vi "Actor Core.vi"(8 "error in":errorcluster caption="错误输入", 11 "Input Operator in":refnum<class "ControlPanel.lvclass"> caption="操作者输入") -> (0 "error out":errorcluster caption="错误输出", 3 "操作者输出":refnum<class "Actor.lvclass">)   [LabVIEW 2014, in "ControlPanel.lvlib" / "ControlPanel.lvclass"]
doc: "(<B>文件名</B>：Actor Framework.lvlib:Actor.lvclass:Actor Core.vi)\n\n接收发送至操作者的消息，响应消息并处理可能导致操作者关闭的错误。\n\n子孙类重写该VI，使操作者完成特定的任务。使用调用父方法节点实现重写。"
uses:
  ControlPanel.lvclass
  <vilib>/ActorFramework/Actor/Actor.lvclass
  ctl/XBOX_Control.ctl
  <vilib>/MakerHub/Xbox-One-Controller/Private/Type Defs/Indicators/All Buttons Visual.ctl
  <vilib>/MakerHub/Xbox-One-Controller/Private/Type Defs/Indicators/A.ctl
  <vilib>/MakerHub/Xbox-One-Controller/Private/Type Defs/Indicators/B.ctl
  <vilib>/MakerHub/Xbox-One-Controller/Private/Type Defs/Indicators/X.ctl
  <vilib>/MakerHub/Xbox-One-Controller/Private/Type Defs/Indicators/Y.ctl
  <vilib>/MakerHub/Xbox-One-Controller/Private/Type Defs/Indicators/Left Bumper.ctl
  <vilib>/MakerHub/Xbox-One-Controller/Private/Type Defs/Indicators/Right Bumper.ctl
  <vilib>/MakerHub/Xbox-One-Controller/Private/Type Defs/Indicators/View.ctl
  <vilib>/MakerHub/Xbox-One-Controller/Private/Type Defs/Indicators/Menu.ctl
  <vilib>/MakerHub/Xbox-One-Controller/Private/Type Defs/Indicators/Thumbstick.ctl
  <vilib>/MakerHub/Xbox-One-Controller/Private/Type Defs/Indicators/All Axis Data.ctl
  <vilib>/MakerHub/Xbox-One-Controller/Private/Type Defs/Indicators/DPad Enum.ctl
  ctl/P3AT_InputCMD.ctl
  ctl/P3AT_Panel.ctl
  ctl/Actor_Control.ctl
  ctl/Semantic_Voice_Array.ctl
  ctl/P3AT_Ini_Pose_send_return.ctl
  JoyStick_lib/JoyStick/JoyStick.lvclass
  Dialogue_lib/DialogueActor/Dialogue.lvclass
  <vilib>/ActorFramework/Actor/Actor.lvclass/Actor.ctl
  <vilib>/ActorFramework/Message Enqueuer/Message Enqueuer.lvclass/Message Enqueuer.ctl
  ControlPanel.lvclass/ControlPanel.ctl
  <vilib>/ActorFramework/Message Enqueuer/Init from Existing Queue.vi
  <vilib>/ActorFramework/Message Enqueuer/Enqueue.vi
  Global_var/Global_var.vi
  <vilib>/ActorFramework/Message Priority Queue/Priority Enqueue.vi
  <vilib>/ActorFramework/Message Enqueuer/Message Enqueuer.lvclass
  Voice_lib/VoiceControl/Voice.lvclass
  <vilib>/ActorFramework/Stop Msg/Stop Msg.lvclass
  Wrapper_lib/zsActor/ActorWrapper.lvclass
  <vilib>/MakerHub/Xbox-One-Controller/LMH-Xbox-One-Controller.lvlib
panel:
  out "Semantic_DialoguePYPL_Array":T1
  out "Semantic_Dialogue_Array":T1
  out "Global_Planner_Recyle":bool
  in  "手动定位":T2
  out "Semantic_Voice_Array":T1
  out "P3AT_InputCMD":T3
  out "XBOX_Control":T4
  out "事件记录":string
  out "sensor":cluster{"voltage":dbl, "motor":i8} {"voltage" scale=0.0..18.0}
  in  "组件管理":T17={"JoyStick"=TRUE, "RemoteP3AT"=TRUE, "DNL_Stop"=FALSE}
  in  "P3AT_Panel":T18={"max_vel"=0.49056603773584906, "max_rot"=0.5094339622641509, "Control_Mode"=enum."Undefined"} {"max_rot" scale=0.0..1.0; "max_vel" scale=0.0..1.0}
  in  "停止信号":bool
  # "下一个版本中加入此功能，文字对话功能，应该设置为枚举值\n最后一个布尔值确认发送"
  # "改变才发送\n所以必须有默认值"
  # "机器人配置信息包括：\n当前线速度；最大线速度；\n当前角速度；最大角速度；\n出生坐标（x,y,rot）；"
  # "此前面板是主要的人机交互界面\n监管者可以使用标准输入设备进行控制\n主要的信息显示将转移到“协调者”和“地图显示器”的前面板"
  # "语音模式操作指南\n在手机上先点“开启广播”，然后再点“获取数据”\n再按“添加语音”"
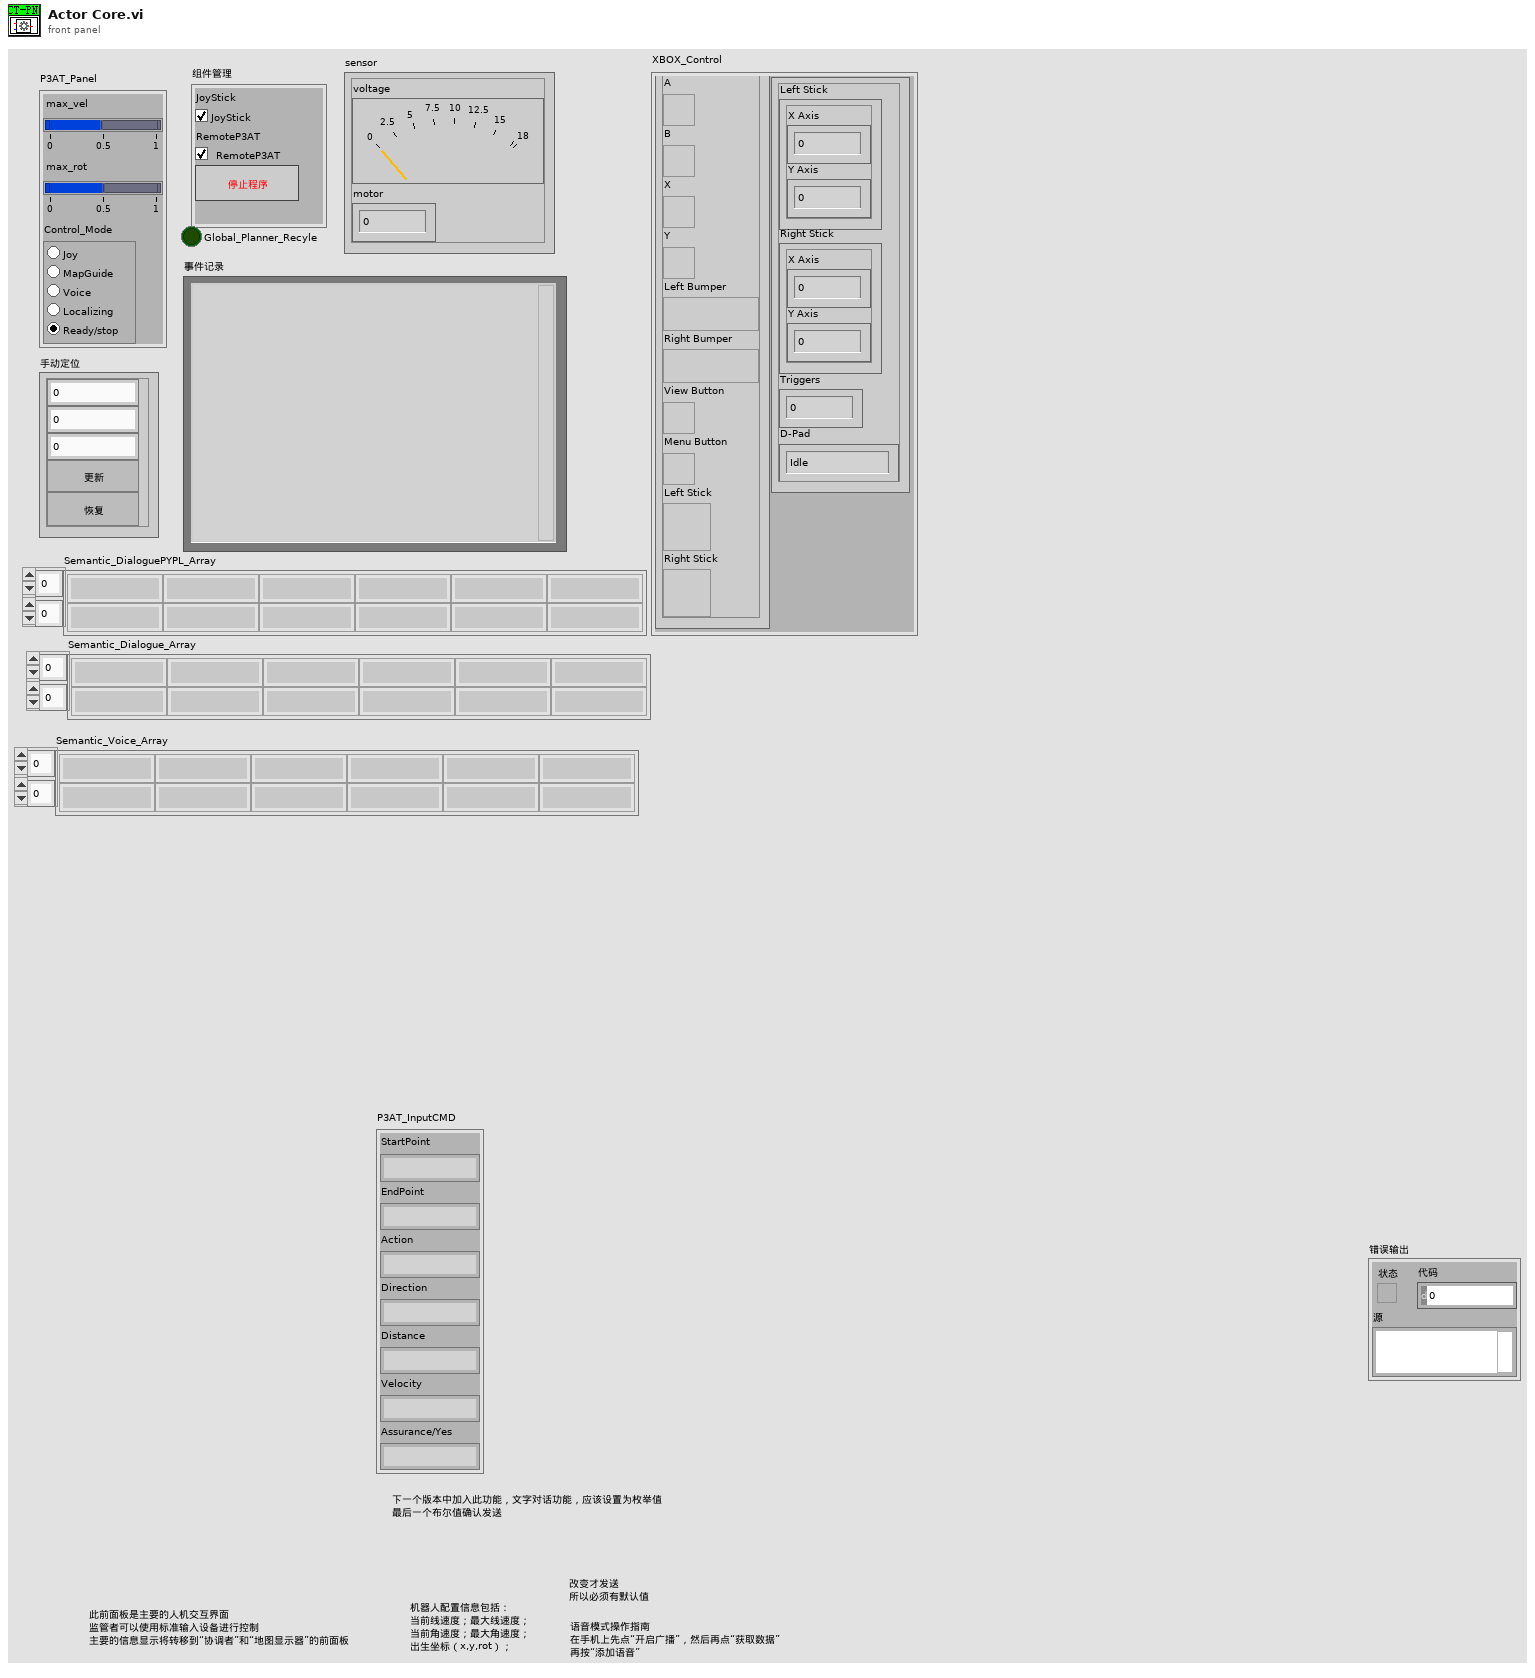
[diagram p1: front panel]
types:
  T1 = typedef "Semantic_Voice_Array.ctl" = string[][]
  T2 = typedef "P3AT_Ini_Pose_send_return.ctl" = cluster{"Ini_pose_X":dbl, "Ini_pose_Y":dbl, "Ini_pose_Rot_deg":dbl, "Send":bool, "Return":bool}
  T3 = typedef "P3AT_InputCMD.ctl" = cluster{"StartPoint":string, "EndPoint":string, "Action":string, "Direction":string, "Distance":string, "Velocity":string, "Assurance/Yes":string}
  T4 = typedef "XBOX_Control.ctl" = cluster{"Buttons":T5, "All Axis":T15}
  T5 = typedef "LMH-Xbox-One-Controller.lvlib/All Buttons Visual.ctl" = cluster{"A":T6, "B":T7, "X":T8, "Y":T9, "Left Bumper":T10, "Right Bumper":T11, "View Button":T12, "Menu Button":T13, "Left Stick":T14, "Right Stick":T14}
  T6 = typedef "LMH-Xbox-One-Controller.lvlib/A.ctl" = bool
  T7 = typedef "LMH-Xbox-One-Controller.lvlib/B.ctl" = bool
  T8 = typedef "LMH-Xbox-One-Controller.lvlib/X.ctl" = bool
  T9 = typedef "LMH-Xbox-One-Controller.lvlib/Y.ctl" = bool
  T10 = typedef "LMH-Xbox-One-Controller.lvlib/Left Bumper.ctl" = bool
  T11 = typedef "LMH-Xbox-One-Controller.lvlib/Right Bumper.ctl" = bool
  T12 = typedef "LMH-Xbox-One-Controller.lvlib/View.ctl" = bool
  T13 = typedef "LMH-Xbox-One-Controller.lvlib/Menu.ctl" = bool
  T14 = typedef "LMH-Xbox-One-Controller.lvlib/Thumbstick.ctl" = bool
  T15 = typedef "LMH-Xbox-One-Controller.lvlib/All Axis Data.ctl" = cluster{"Left Stick":cluster{"X Axis":i32, "Y Axis":i32}, "Right Stick":cluster{"X Axis":i32, "Y Axis":i32}, "Triggers":i32, "D-Pad":T16}
  T16 = typedef "LMH-Xbox-One-Controller.lvlib/DPad Enum.ctl" = enum16{"Idle", "Up", "Up / Right", "Right", "Down / Right", "Down", "Down / Left", "Left", "Up / Left"}
  T17 = typedef "Actor_Control.ctl" = cluster{"JoyStick":bool, "RemoteP3AT":bool, "DNL_Stop":bool}
  T18 = typedef "P3AT_Panel.ctl" = cluster{"max_vel":dbl, "max_rot":dbl, "Control_Mode":enum32{"Joy", "Map", "Voice", "Input", "Undefined"}}
  T19 = enum32{"Joy", "Map", "Voice", "Input", "Undefined"}
  T20 = cluster{"Ini_pose_X":dbl, "Ini_pose_Y":dbl, "Ini_pose_Rot_deg":dbl}
  T21 = typedef "P3AT_Current.ctl" = cluster{"max_vel":dbl, "max_rot":dbl, "now_pose_X":dbl, "now_pose_Y":dbl, "now_pose_Rot_deg":dbl, "Control_Mode":enum32{"Joy", "Map", "Voice", "Input", "Undefined"}}
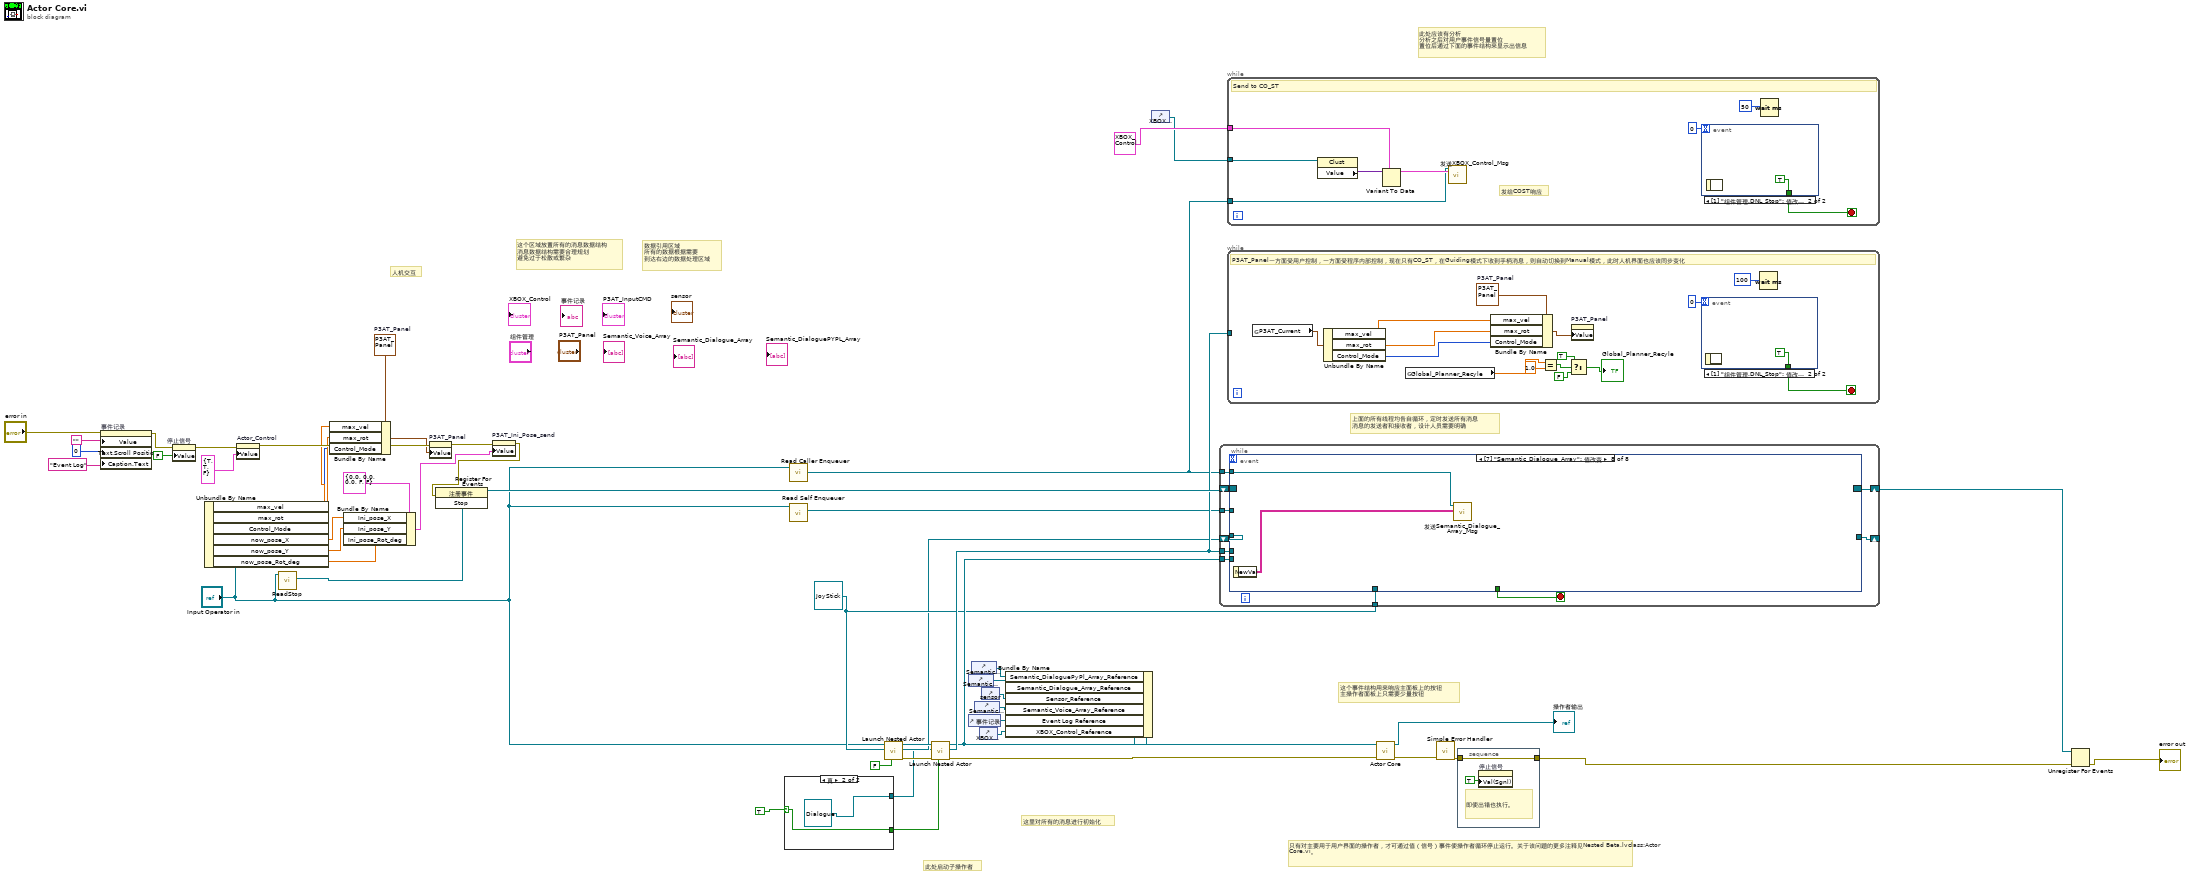
[diagram p0: block diagram]
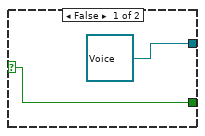
[diagram p2: hidden frame]
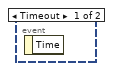
[diagram p3: hidden frame]
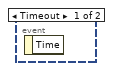
[diagram p4: hidden frame]
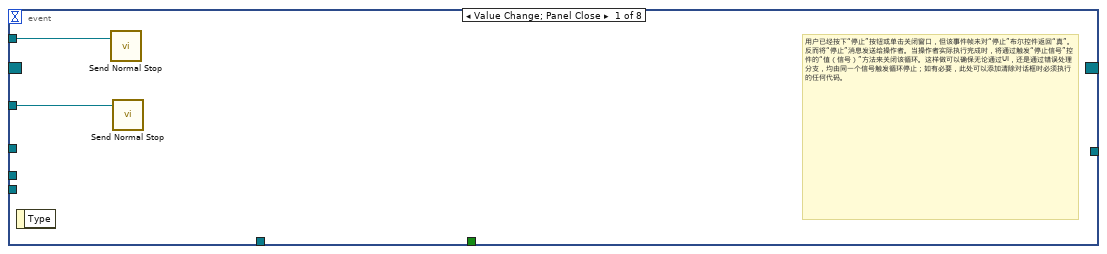
[diagram p5: hidden frame]
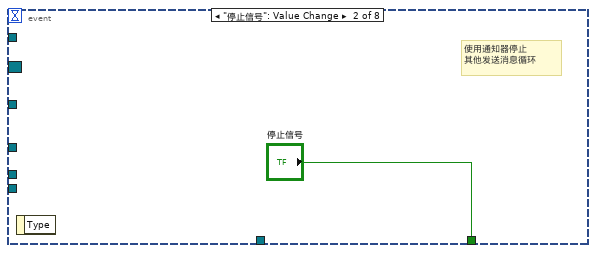
[diagram p6: hidden frame]
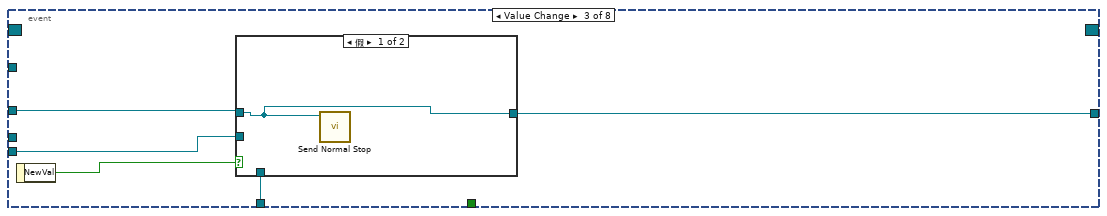
[diagram p7: hidden frame]
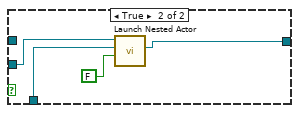
[diagram p8: hidden frame]
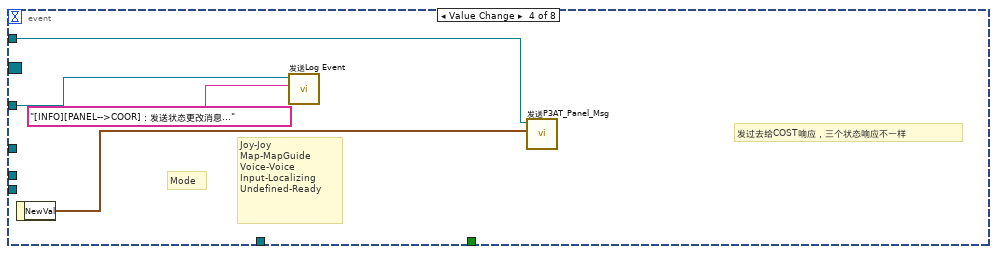
[diagram p9: hidden frame]
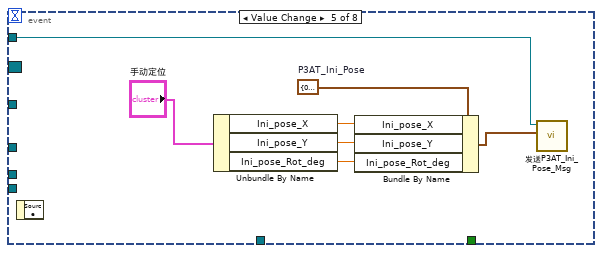
[diagram p10: hidden frame]
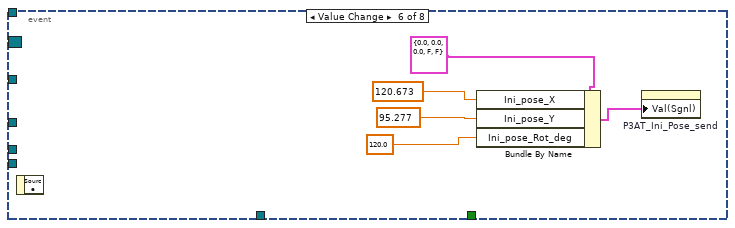
[diagram p11: hidden frame]
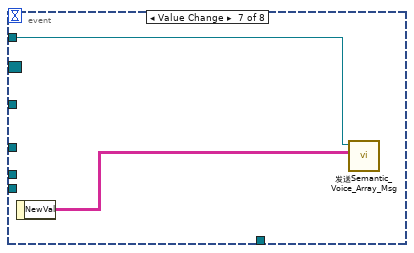
[diagram p12: hidden frame]
diagram:
  w24 = T18 {"max_vel"=0.49056603773584906, "max_rot"=0.5094339622641509, "Control_Mode"=enum."Joy"}  # P3AT_Panel
  w27 = refnum<class "JoyStick.lvclass"> refnum ("JoyStick.lvlib:JoyStick.lvclass")
  # "人机交互"
  # "此处应该有分析\n分析之后对用户事件信号量置位\n置位后通过下面的事件结构来显示出信息"
  # "这里对所有的消息进行初始化"
  # "此处启动子操作者"
  # "数据引用区域\n所有的数据根据需要\n到达右边的数据处理区域"
  # "这个区域放置所有的消息数据结构\n消息数据结构需要合理规划\n避免过于松散或繁杂"
  # "这个事件结构用来响应主面板上的按钮\n主操作者面板上只需要少量按钮"
  # "上面的所有线程均各自循环，定时发送所有消息\n消息的发送者和接收者，设计人员需要明确"
  # "只有对主要用于用户界面的操作者，才可通过值（信号）事件使操作者循环停止运行。关于该问题的更多注释见Nested Beta.lvclass:Actor Core.vi。"
  n1 = property on="事件记录" class="Str"(error in="error in", "Value"="", "Text.Scroll Position"=u32 0, "Caption.Text"="Event Log" ("Unlocalized")) -> (error out=w38:errorcluster)  [unwired: 1 in, 1 out]
  n2 = property on="停止信号" class="Bool (严格)"(error in=w38, "Value"=FALSE ("stop")) -> (error out=w30:errorcluster)  [unwired: 1 in, 1 out]
  n3 = Unbundle By Name("Input Operator in") -> ("max_vel"=w23:dbl, "max_rot"=w22:dbl, "Control_Mode"=w21:T19, "now_pose_X"=w13:dbl, "now_pose_Y"=w12:dbl, "now_pose_Rot_deg"=w11:dbl)
  n4 = property on="Actor_Control" class="Clust"(error in=w30, "Value"=T17 {"JoyStick"=TRUE, "RemoteP3AT"=TRUE, "DNL_Stop"=FALSE} ("Actor_Control 2")) -> (error out=w25:errorcluster)  [unwired: 1 in, 1 out]
  n5 = call-dynamic "ReadStop.vi"("zsActor输入"="Input Operator in") -> ("Stop"=w18:refnum<user-event>)  [unwired: 8 in, 2 out]
  n6 = Bundle By Name(cluster=w24, "max_vel"=w23, "max_rot"=w22, "Control_Mode"=w21) -> (w20:T18)
  n7 = Bundle By Name(cluster=T2 {"Ini_pose_X"=0.0, "Ini_pose_Y"=0.0, "Ini_pose_Rot_deg"=0.0, "Send"=FALSE, "Return"=FALSE} ("值(信号)"), "Ini_pose_X"=w13, "Ini_pose_Y"=w12, "Ini_pose_Rot_deg"=w11) -> (w8:T2)
  n8 = property on="P3AT_Panel" class="Clust (严格)"(error in=w25, "Value"=w20) -> (error out=w9:errorcluster)  [unwired: 1 in, 1 out]
  n9 = property on="P3AT_Ini_Pose_send" class="Clust"(error in=w9, "Value"=w8) -> (error out=w7:errorcluster)  [unwired: 1 in, 1 out]
  n10 = register-events(error in=w7, w18) -> (reference out=w42:refnum<event-registration>)  [unwired: 1 in, 1 out]
  n11 = case shown="真" TRUE {
    selector: TRUE -> [w54 w56]
    tunnel: [w54 w56] -> w3
    tunnel: [refnum<class "Voice.lvclass"> refnum ("Voice.lvlib:Voice.lvclass") refnum<class "Dialogue.lvclass"> refnum ("Dialogue.lvlib:Dialogue.lvclass")] -> w4
    frame False {
    }
    frame True {
    }
  }
  n12 = call <vilib>:"Read Caller Enqueuer.vi"("Actor"="Input Operator in") -> ("Caller Enqueuer"=w31:refnum<class "Message Enqueuer.lvclass">)  [unwired: 10 in]
  n13 = call <vilib>:"Read Self Enqueuer.vi"("Actor"="Input Operator in") -> ("Self Enqueuer"=w32:refnum<class "Message Enqueuer.lvclass">)  [unwired: 10 in]
  n14 = call <vilib>:"Launch Nested Actor.vi"("Open Actor Core front panel? (F)"=FALSE, "Nested Actor"=w27, "Caller Actor in"="Input Operator in") -> ("error out"=w51:errorcluster, "Nested Actor's Enqueuer"=w26:refnum<class "Message Enqueuer.lvclass">, "Caller Actor out"=w39:refnum<class "ControlPanel.lvclass">)  [unwired: 6 in]
  n15 = call <vilib>:"Launch Nested Actor.vi"("Open Actor Core front panel? (F)"=w3, "error in (no error)"=w51, "Nested Actor"=w4, "Caller Actor in"=w39) -> ("error out"=w50:errorcluster, "Nested Actor's Enqueuer"=w37:refnum<class "Message Enqueuer.lvclass">, "Caller Actor out"=w28:refnum<class "ControlPanel.lvclass">)  [unwired: 5 in]
  n16 = control-ref of="Semantic_Dialogue_Array"() -> (w2:refnum<vi>)
  n17 = control-ref of="事件记录"() -> (w48:refnum<vi>)
  n18 = control-ref of="Semantic_DialoguePYPL_Array"() -> (w1:refnum<vi>)
  n19 = control-ref of="Semantic_Voice_Array"() -> (w17:refnum<vi>)
  n20 = control-ref of="XBOX_Control"() -> (w36:refnum<vi>)
  n21 = control-ref of="sensor"() -> (w14:refnum<vi>)
  n22 = Bundle By Name(cluster=w28, "Semantic_DialoguePyPl_Array_Reference"=w1, "Semantic_Dialogue_Array_Reference"=w2, "Sensor_Reference"=w14, "Semantic_Voice_Array_Reference"=w17, "Event Log Reference"=w48, "XBOX_Control_Reference"=w36) -> (w49:refnum<class "ControlPanel.lvclass">)
  n23 = control-ref of="XBOX_Control"() -> (w15:refnum<vi>)
  n24 = while {
    tunnel: w31 -> [w66]
    tunnel: w37 -> [w62]
    shift-right: [w63] -> w41
    shift-left: w42 -> [w64]
    tunnel: w32 -> [w61]
    tunnel: w28 -> [w60]
    tunnel: w27 -> [w59]
    shift-right: [w58] -> _
    shift-left: w26 -> [w57]
    stop <- w65 stop-if-true
    n25 = event shown="[7] \"Semantic_Dialogue_Array\": 值改变" {
      selector: w64 -> [_ _ _ _ _ _ _ _]
      dyn-events: [_ _ _ _ _ _ _ _] -> w63
      timeout: _ -> [_ _ _ _ _ _ _ _]
      tunnel: w66 -> [w67 _ _ w83 w90 _ w96 w99]
      tunnel: w62 -> [_ _ _ _ _ _ _ _]
      tunnel: [_ "停止信号" _ _ _ _ _ _] -> w65
      tunnel: w61 -> [w68 _ _ w81 _ _ _ _]
      tunnel: w60 -> [_ _ w73 _ _ _ _ _]
      tunnel: w59 -> [_ _ w72 _ _ _ _ _]
      tunnel: [_ _ w71 _ _ _ _ _] -> w58
      tunnel: w57 -> [_ _ w70 _ _ _ _ _]
      event Value Change; Panel Close {
        # "用户已经按下“停止”按钮或单击关闭窗口，但该事件帧未对“停止”布尔控件返回“真”。反而将“停止”消息发送给操作者。当操作者实际执行完成时，将通过触发“停止信号”控件的“值（信号）”方法来关闭该循环。这样做可以确保无论通过UI，还是通过错误处理分支，均由同一个信号触发循环停止；如有必要，此处可以添加清除对话框时必须执行的任何代码。"
        n26 = event-data() -> ()  [unwired: 1 in, 1 out]
        n27 = call <vilib>:"Send Normal Stop.vi"("Message Enqueuer"=w67) -> ()  [unwired: 10 in, 1 out]
        n28 = call <vilib>:"Send Normal Stop.vi"("Message Enqueuer"=w68) -> ()  [unwired: 10 in, 1 out]
      }
      event "停止信号": Value Change {
        # "使用通知器停止\n其他发送消息循环"
        n29 = event-data() -> ()  [unwired: 1 in, 1 out]
      }
      event Value Change {
        n30 = event-data() -> ("NewVal"=w74:bool)  [unwired: 1 in]
        n31 = case shown="假" w74 {
          tunnel: w73 -> [_ w78]
          tunnel: w72 -> [_ w77]
          tunnel: [w75 w76] -> w71
          tunnel: w70 -> [w75 _]
          frame False {
            n32 = call <vilib>:"Send Normal Stop.vi"("Message Enqueuer"=w75) -> ()  [unwired: 10 in, 1 out]
          }
          frame True {
            n33 = call <vilib>:"Launch Nested Actor.vi"("Auto-stop? (T)"=FALSE ("Open Actor Core front panel? (F)"), "Nested Actor"=w77, "Caller Actor in"=w78) -> ("Nested Actor's Enqueuer"=w76:refnum<class "Message Enqueuer.lvclass">)  [unwired: 6 in, 2 out]
          }
        }
      }
      event Value Change {
        # "Mode"
        # "Joy-Joy\nMap-MapGuide\nVoice-Voice\nInput-Localizing\nUndefined-Ready"
        # "发过去给COST响应，三个状态响应不一样"
        n34 = event-data() -> ("NewVal"=w82:T18)  [unwired: 1 in]
        n35 = call "发送Log Event.vi"("Event Text"="[INFO][PANEL-->COOR]：发送状态更改消息...", "消息待入队列"=w81) -> ()  [unwired: 8 in, 2 out]
        n36 = call "发送P3AT_Panel_Msg.vi"("值(信号)"=w82, "消息待入队列"=w83) -> ()  [unwired: 8 in, 2 out]
      }
      event Value Change {
        w88 = T20 {"Ini_pose_X"=0.0, "Ini_pose_Y"=0.0, "Ini_pose_Rot_deg"=0.0}  # P3AT_Ini_Pose
        n37 = event-data() -> ()  [unwired: 1 in, 1 out]
        n38 = Unbundle By Name("手动定位") -> ("Ini_pose_X"=w87:dbl, "Ini_pose_Y"=w86:dbl, "Ini_pose_Rot_deg"=w85:dbl)
        n39 = Bundle By Name(cluster=w88, "Ini_pose_X"=w87, "Ini_pose_Y"=w86, "Ini_pose_Rot_deg"=w85) -> (w84:T20)
        n40 = call "发送P3AT_Ini_Pose_Msg.vi"("值(信号)"=w84, "消息待入队列"=w90) -> ()  [unwired: 8 in, 2 out]
      }
      event Value Change {
        n41 = event-data() -> ()  [unwired: 1 in, 1 out]
        n42 = Bundle By Name(cluster=T2 {"Ini_pose_X"=0.0, "Ini_pose_Y"=0.0, "Ini_pose_Rot_deg"=0.0, "Send"=FALSE, "Return"=FALSE} ("值(信号)"), "Ini_pose_X"=120.673, "Ini_pose_Y"=95.277, "Ini_pose_Rot_deg"=120.0) -> (w95:T2)
        n43 = property on="P3AT_Ini_Pose_send" class="Clust"("Val(Sgnl)"=w95) -> ()  [unwired: 2 in, 2 out]
      }
      event Value Change {
        n44 = event-data() -> ("NewVal"=w97:T1)  [unwired: 1 in]
        n45 = call "发送Semantic_Voice_Array_Msg.vi"("值(信号)"=w97, "消息待入队列"=w96) -> ()  [unwired: 8 in, 2 out]
      }
      event Value Change {
        n46 = event-data() -> ("NewVal"=w98:T1)  [unwired: 1 in]
        n47 = call "发送Semantic_Dialogue_Array_Msg.vi"("值(信号)"=w98, "消息待入队列"=w99) -> ()  [unwired: 8 in, 2 out]
      }
    }
  }
  n48 = while {
    tunnel: w37 -> [_]
    stop <- w112 stop-if-true
    w109 = T18 {"max_vel"=0.49056603773584906, "max_rot"=0.5094339622641509, "Control_Mode"=enum."Joy"}  # P3AT_Panel
    # "P3AT_Panel一方面受用户控制，一方面受程序内部控制，现在只有CO_ST，在Guiding模式下收到手柄消息，则自动切换到Manual模式，此时人机界面也应该同步变化"
    n49 = global read "Global_var.vi" "P3AT_Current"() -> (w111:T21)
    n50 = Unbundle By Name(w111) -> ("max_vel"=w108:dbl, "max_rot"=w107:dbl, "Control_Mode"=w106:T19)
    n51 = global read "Global_var.vi" "Global_Planner_Recyle"() -> (w101:dbl)
    n52 = Bundle By Name(cluster=w109, "max_vel"=w108, "max_rot"=w107, "Control_Mode"=w106) -> (w110:T18)
    n53 = Equal?(x=w101, y=1.0) -> (x = y?=w104:bool)
    n54 = Select(t=TRUE, s=w104, f=FALSE) -> (s? t:f=→"Global_Planner_Recyle":bool)
    n55 = property on="P3AT_Panel" class="Clust (严格)"("Value"=w110) -> ()  [unwired: 2 in, 2 out]
    n56 = event shown="[1] \"组件管理.DNL_Stop\": 值改变" {
      selector: _ -> [_ _]
      dyn-events: _ -> [_ _]
      timeout: 0 -> [_ _]
      tunnel: [_ TRUE] -> w112
      event Timeout {
        n57 = event-data() -> ()  [unwired: 1 in, 1 out]
      }
      event Value Change {
        n58 = event-data() -> ()  [unwired: 1 in, 1 out]
      }
    }
    n59 = Wait (ms)(milliseconds to wait=u32 100 ("等待时间（毫秒）")) -> ()  [unwired: 1 out]
  }
  n60 = while {
    tunnel: w31 -> [w116]
    tunnel: T4 {"Buttons"={"A"=FALSE, "B"=FALSE, "X"=FALSE, "Y"=FALSE, "Left Bumper"=FALSE, "Right Bumper"=FALSE, "View Button"=FALSE, "Menu Button"=FALSE, "Left Stick"=FALSE, "Right Stick"=FALSE}, "All Axis"={"Left Stick"={"X Axis"=0, "Y Axis"=0}, "Right Stick"={"X Axis"=0, "Y Axis"=0}, "Triggers"=0, "D-Pad"=enum."Idle"}} ("XBOX_Control 2") -> [w119]
    tunnel: w15 -> [w118]
    stop <- w121 stop-if-true
    # "发给COST响应"
    # "Send to CO_ST"
    n61 = property class="Clust"(reference=w118) -> ("Value"=w120:variant)  [unwired: 1 in, 2 out]
    n62 = Variant To Data(type=w119, Variant=w120) -> (data=w117:T4)  [unwired: 1 in, 1 out]
    n63 = call "发送XBOX_Control_Msg.vi"("XBOX_Control"=w117, "消息待入队列"=w116) -> ()  [unwired: 8 in, 2 out]
    n64 = event shown="[1] \"组件管理.DNL_Stop\": 值改变" {
      selector: _ -> [_ _]
      dyn-events: _ -> [_ _]
      timeout: 0 -> [_ _]
      tunnel: [_ TRUE] -> w121
      event Timeout {
        n65 = event-data() -> ()  [unwired: 1 in, 1 out]
      }
      event Value Change {
        n66 = event-data() -> ()  [unwired: 1 in, 1 out]
      }
    }
    n67 = Wait (ms)(milliseconds to wait=u32 50 ("等待时间（毫秒）")) -> ()  [unwired: 1 out]
  }
  n68 = call-parent "Actor Core.vi"("error in"=w50, "Actor in"=w49) -> ("error out"=w44:errorcluster, "Actor out"=→"操作者输出":refnum<class "Actor.lvclass">)  [unwired: 8 in]
  n69 = call <vilib>:"Simple Error Handler.vi"("error in (no error)"=w44) -> ("error out"=w43:errorcluster)  [unwired: 4 in, 4 out]
  n70 = stacked-sequence {
    tunnel: [w125] -> w40
    tunnel: w43 -> [w125]
    frame #0 {
      # "即使出错也执行。"
      n71 = property on="停止信号" class="Bool (严格)"("Val(Sgnl)"=TRUE ("stop")) -> ()  [unwired: 2 in, 2 out]
    }
  }
  n72 = Unregister For Events(event registration refnum=w41, error in=w40) -> (error out=→"error out":errorcluster)
